vi "MEMR-Plot IO.vi"(0 "Metrics":dbl[][](array[numeric]), 1 "IO":refnum<vi>, 5 "Level":dbl[](array[numeric]), 7 "Threshold":dbl, 9 "Noise metrics":dbl[](array[numeric]), 11 "error in (no error)":errorcluster, 12 "Criterion":dbl) -> (15 "error out":errorcluster)   [LabVIEW 2020]
uses:
  <vilib>/Analysis/baseanly.llb/Mean (DBL).vi
  <vilib>/Analysis/NI_AALBase.lvlib
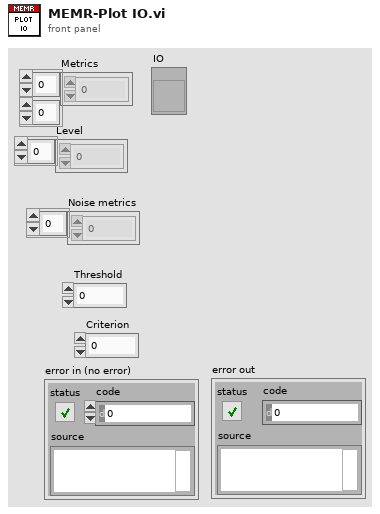
[diagram p1: front panel]
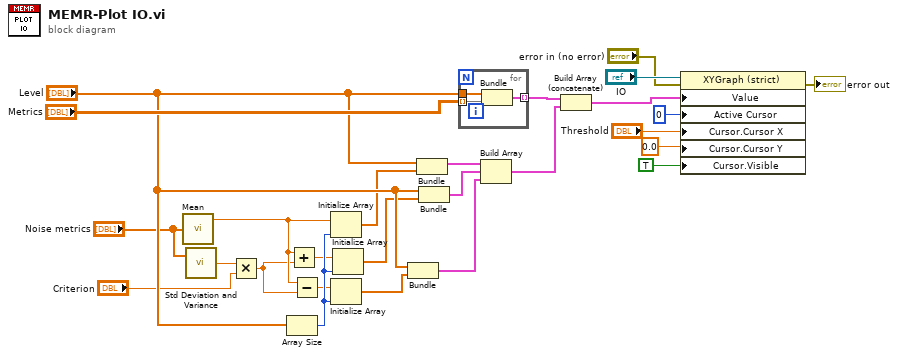
[diagram p0: block diagram]
diagram:
  n1 = call-poly <vilib>:"Mean.vi"("X"="Noise metrics") -> ("mean"=w10:dbl)  [unwired: 1 out]
  n2 = call <vilib>:"Std Deviation and Variance.vi"("X"="Noise metrics") -> ("standard deviation"=w11:dbl)  [unwired: 1 in, 2 out]
  n3 = Multiply(x=w11, y="Criterion") -> (x*y=w2:dbl)
  n4 = Array Size(array="Level") -> (size(s)=w13:i32)
  n5 = Add(x=w10, y=w2) -> (x+y=w9:dbl)
  n6 = Subtract(x=w10, y=w2) -> (x-y=w12:dbl)
  n7 = Initialize Array(w10, w13) -> (w6:dbl[])
  n8 = Initialize Array(w12, w13) -> (w8:dbl[])
  n9 = Initialize Array(w9, w13) -> (w7:dbl[])
  n10 = Bundle("Level"="Level", w8) -> (w16:cluster{"Level":dbl[], dbl[]})  [unwired: 1 in]
  n11 = Bundle("Level"="Level", w6) -> (w14:cluster{"Level":dbl[], dbl[]})  [unwired: 1 in]
  n12 = Bundle("Level"="Level", w7) -> (w15:cluster{"Level":dbl[], dbl[]})  [unwired: 1 in]
  n13 = for {
    tunnel: "Metrics" -> [w29] mode=indexing
    tunnel: [w28] -> w23 mode=indexing
    tunnel: "Level" -> [w27]
    n14 = Bundle("Level"=w27, "Metrics"=w29) -> (w28:cluster{"Level":dbl[], "Metrics":dbl[]})  [unwired: 1 in]
  }
  n15 = Build Array(w14, w15, w16) -> (w3:cluster{"Level":dbl[], dbl[]}[])
  n16 = Build Array (concatenate)(w23, w3) -> (w4:cluster{"Level":dbl[], "Metrics":dbl[]}[])
  n17 = property on="Property Node" class="XYGraph (strict)"(reference="IO", error in="error in (no error)", "Value"=w4, "Active Cursor"=u32 0, "Cursor.Cursor X"="Threshold", "Cursor.Cursor Y"=0.0 ("Cursor.Cursor Position:Cursor Y"), "Cursor.Visible"=TRUE) -> (error out=→"error out":errorcluster)  [unwired: 1 out]
